vi "main.vi"() -> ()   [LabVIEW 2020]
doc: "This VI is used to talk with the psrr device and handle the errors produced by it."
uses:
  Typedef's/Last_Error_Details.ctl
  Typedef's/Q_Operations.ctl
  Typedef's/Q_State.ctl
  Typedef's/User_Events_Operations.ctl
  Typedef's/Data_Cluster.ctl
  Typedef's/Timer_Operations.ctl
  Typedef's/Error_Cluster.ctl
  Typedef's/PSRR_Value.ctl
  Typedef's/Error_Count.ctl
  Typedef's/Constants.ctl
  <vilib>/SLL Toolkit/SLL String/_SubVIs/I32 to String.vi
  <vilib>/SLL Toolkit/SLL String/SLL String.lvlib
panel:
  out "Last Error Details":T1
  out "Obtained PSRR":i32(graph)
  out "Table":string[][](table)
  in  "Error Log":bool
  out "Last Read PSRR (dB)":i32
  in  "Exit":bool
  in  "Wait Time (sec)":dbl=2.0 min=2.0
  out "Error?":bool
  out "Error Out":errorcluster
  in  "Error In":errorcluster
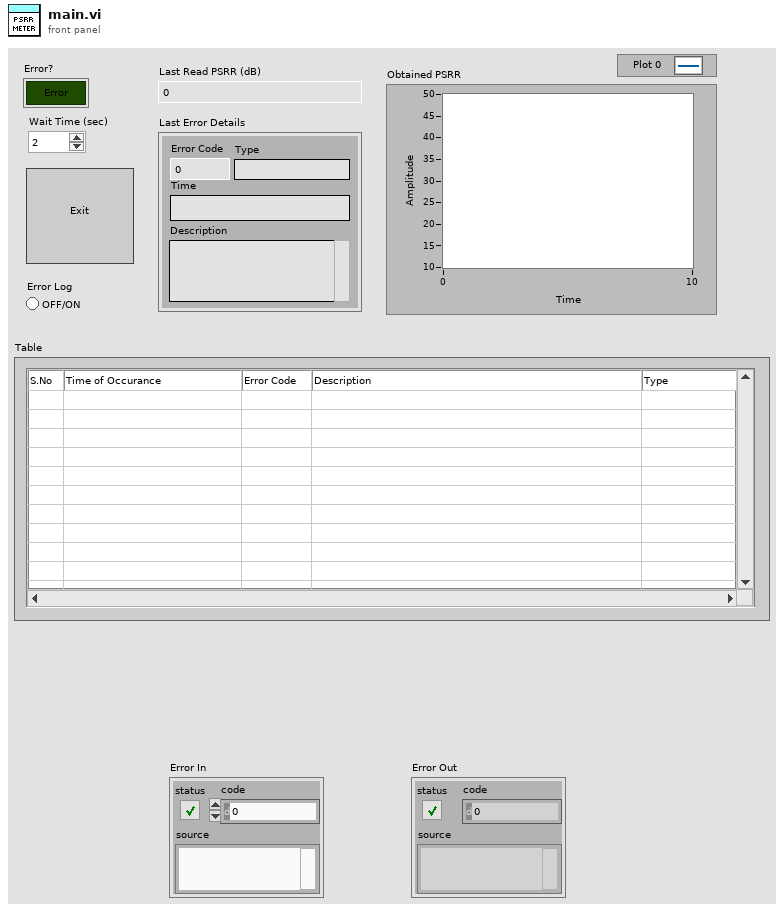
[diagram p1: front panel]
types:
  T1 = typedef "Last_Error_Details.ctl" = cluster{"Description":string, "Time":string, "Error Code":i32, "Type":string}
  T2 = typedef "Q_Operations.ctl" = enum16{"Create Q", "Enqueue", "Dequeue", "Enqueue N ele", "Enstack N ele", "Flush Q", "Destroy Q"}
  T3 = typedef "User_Events_Operations.ctl" = enum16{"Create", "Generate", "Destroy"}
  T4 = typedef "Q_State.ctl" = cluster{"State":string, "Data":variant}
  T5 = typedef "Data_Cluster.ctl" = cluster{"Wait Time":dbl, "Timer Operations":T6, "Error":T7, "Last Error Details":T1, "PSRR Value":T8, "Table Data":string[][], "Error Log?":bool, "Count":T9, "Constants":T10, "Data Folder Path":path}
  T6 = typedef "Timer_Operations.ctl" = cluster{"Prev Time":timestamp, "Set Time":timestamp}
  T7 = typedef "Error_Cluster.ctl" = errorcluster
  T8 = typedef "PSRR_Value.ctl" = cluster{"PSRR dB":i32, "PSRR Value Update?":bool}
  T9 = typedef "Error_Count.ctl" = cluster{"Passive Error":u8, "Unknown Error":u8, "S. No":i32}
  T10 = typedef "Constants.ctl" = cluster{"No Of Error":u8}
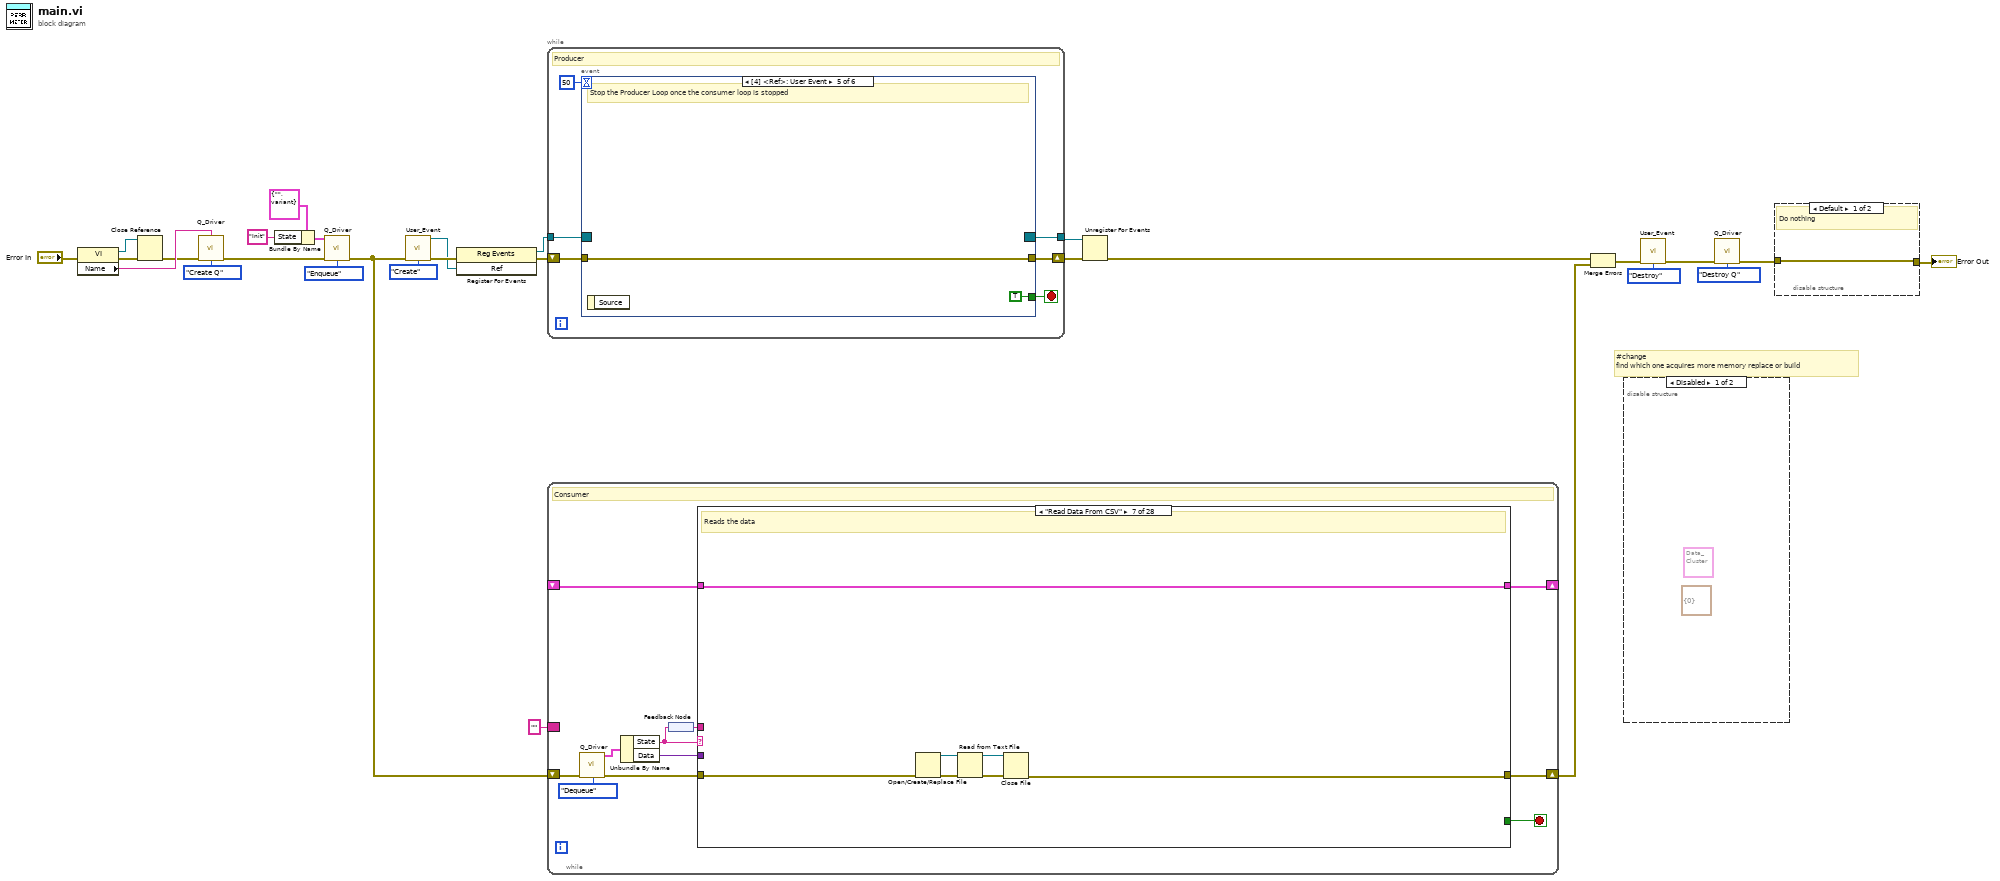
[diagram p0: block diagram]
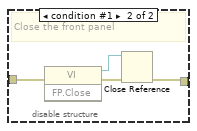
[diagram p3: hidden frame]
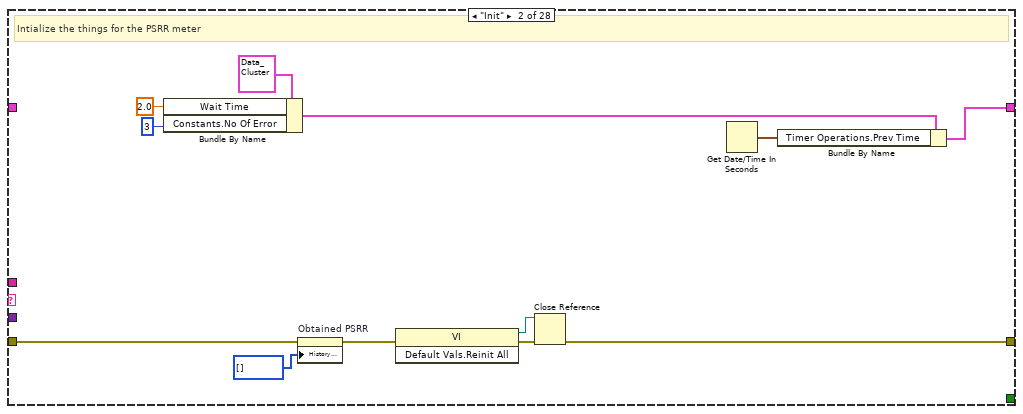
[diagram p5: hidden frame]
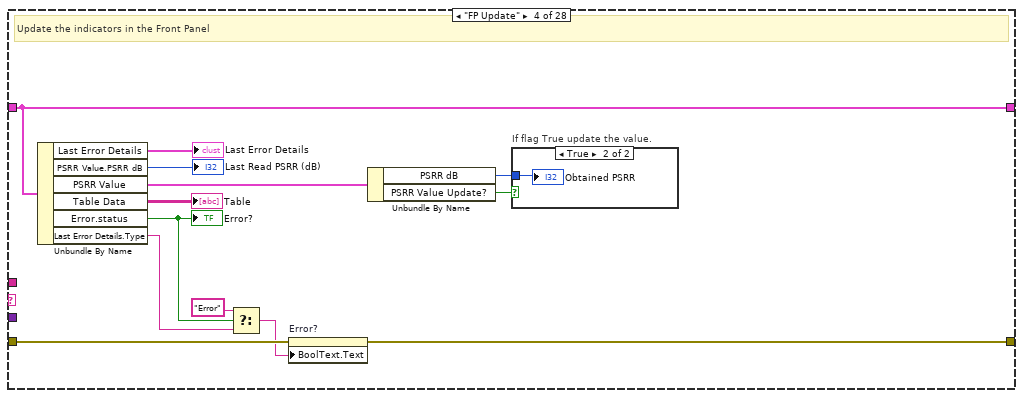
[diagram p7: hidden frame]
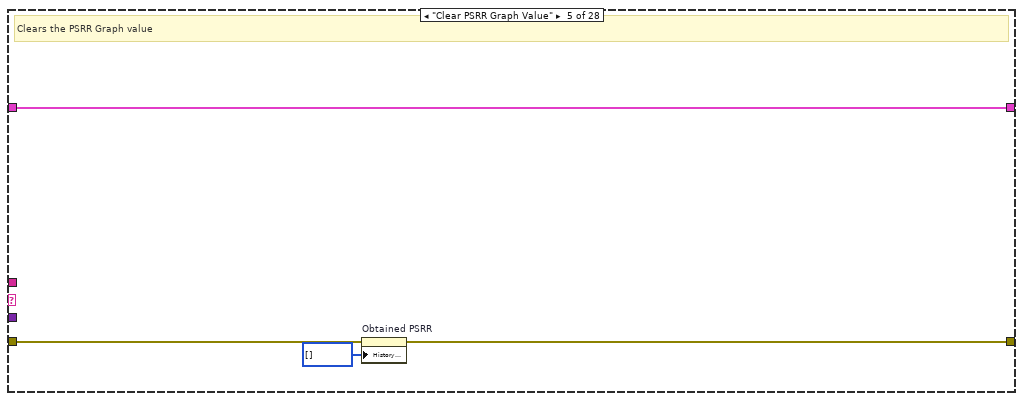
[diagram p9: hidden frame]
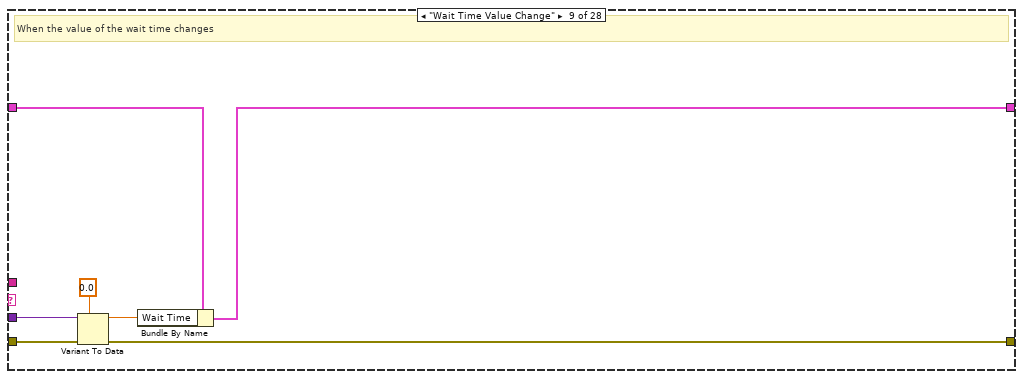
[diagram p12: hidden frame]
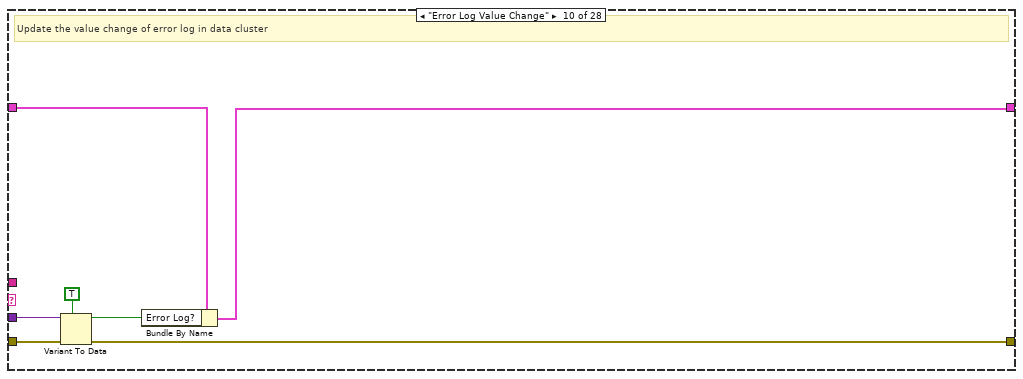
[diagram p13: hidden frame]
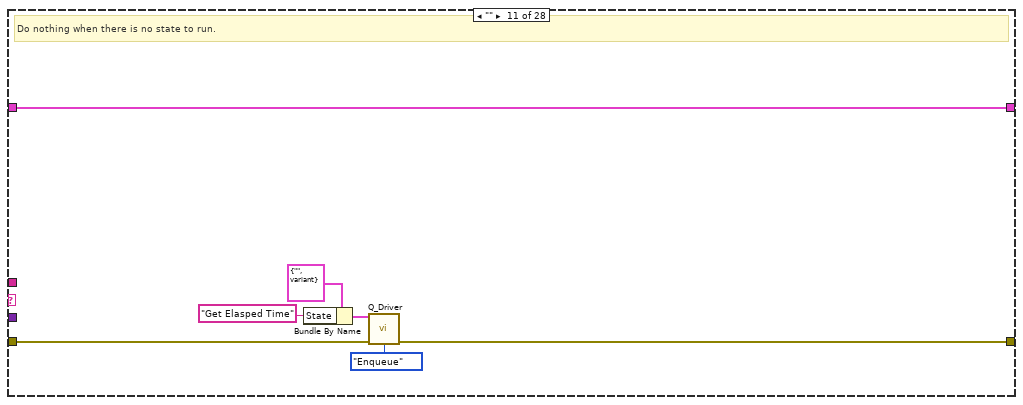
[diagram p14: hidden frame]
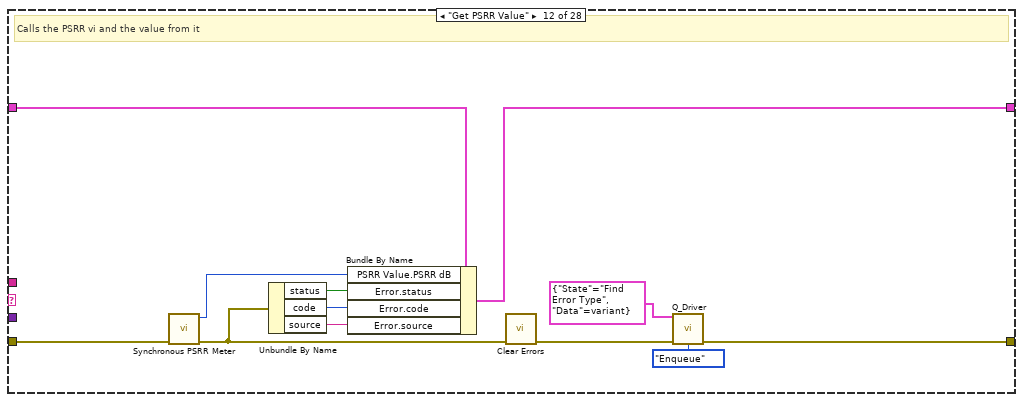
[diagram p15: hidden frame]
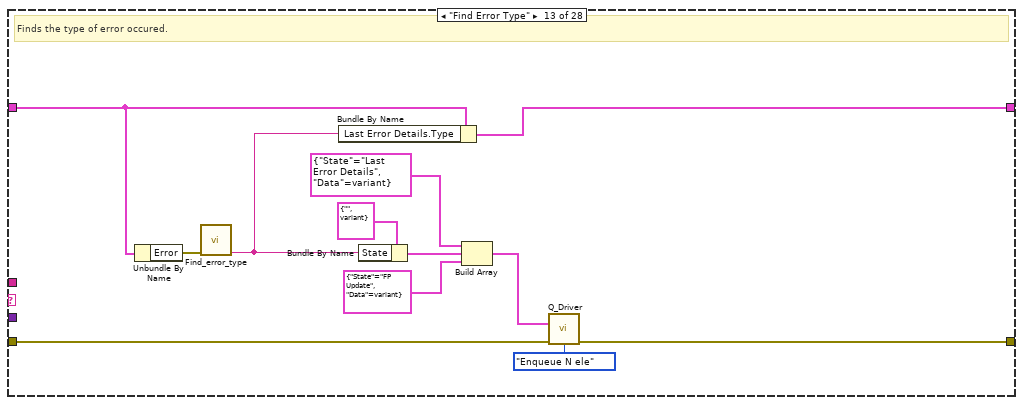
[diagram p16: hidden frame]
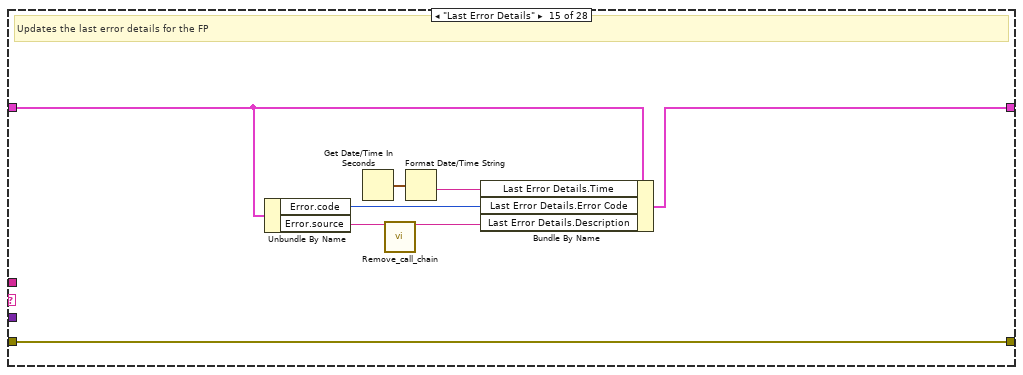
[diagram p18: hidden frame]
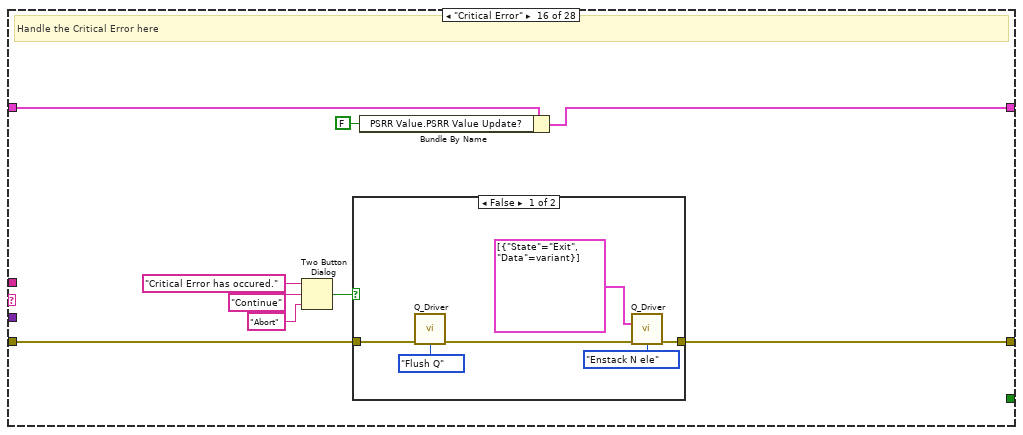
[diagram p19: hidden frame]
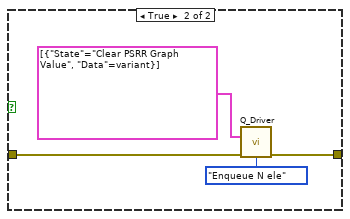
[diagram p20: hidden frame]
diagram:
  # "#change\nfind which one acquires more memory replace or build"
  n1 = property class="VI"(error in="Error In") -> (reference out=w5:refnum<vi>, error out=w24:errorcluster, "Name"=w23:string)  [unwired: 1 in]
  n2 = Close Reference(reference=w5, error in (no error)=w24) -> (error out=w21:errorcluster)
  n3 = call "Q_Driver.vi"("Q_Name"=w23, "Error In"=w21, "Operations"=Q_Operations."Create Q") -> ("Error Out"=w20:errorcluster)  [unwired: 11 in, 1 out]
  n4 = Bundle By Name(cluster=T4 {"State"="", "Data"=variant} ("State"), "State"="Init") -> (w15:T4)
  n5 = call "Q_Driver.vi"("State"=w15, "Error In"=w20, "Operations"=Q_Operations."Enqueue") -> ("Error Out"=w19:errorcluster)  [unwired: 11 in, 1 out]
  n6 = call "User_Event.vi"("Error In"=w19, "Enum"=User_Events_Operations."Create") -> ("Ref"=w11:refnum<user-event>, "Error Out"=w14:errorcluster)  [unwired: 12 in]
  n7 = register-events(error in=w14, w11) -> (reference out=w10:refnum<event-registration>, error out=w12:errorcluster)  [unwired: 1 in]
  n8 = while {
    shift-right: [w31] -> w28
    shift-left: w12 -> [w32]
    tunnel: w10 -> [w30]
    tunnel: [w29] -> w8
    stop <- w33 stop-if-true
    # "Producer"
    n9 = event shown="[4] <Ref>: User Event" {
      selector: w30 -> [_ _ _ _ _ _]
      dyn-events: [_ _ _ _ _ _] -> w29
      timeout: 50 -> [_ _ _ _ _ _]
      tunnel: [_ _ _ _ TRUE _] -> w33
      tunnel: w32 -> [w35 w36 w50 w55 w57 w58]
      tunnel: [w35 w43 w51 w54 w57 w59] -> w31
      event Timeout {
        # "When there is no event triggered."
        n10 = event-data() -> ()  [unwired: 1 in, 1 out]
      }
      event "Error Log": Value Change {
        # "When the error log is turned on"
        n11 = event-data() -> ("NewVal"=w39:bool)  [unwired: 1 in]
        n12 = To Variant(anything=w39) -> (Variant=w38:variant)
        n13 = Bundle By Name(cluster=T4 {"State"="", "Data"=variant} ("State"), "State"="Error Log Value Change", "Data"=w38) -> (w37:T4)
        n14 = call "Q_Driver.vi"("State"=w37, "Error In"=w36, "Operations"=Q_Operations."Enqueue") -> ("Error Out"=w43:errorcluster)  [unwired: 11 in, 1 out]
      }
      event "Wait Time (sec)": Value Change {
        # "When there is value change for error creation."
        n15 = event-data() -> ("NewVal"=w47:dbl)  [unwired: 1 in]
        n16 = To Variant(anything=w47) -> (Variant=w46:variant)
        n17 = Bundle By Name(cluster=T4 {"State"="", "Data"=variant} ("State"), "State"="Wait Time Value Change", "Data"=w46) -> (w44:T4)
        n18 = call "Q_Driver.vi"("State"=w44, "Error In"=w50, "Operations"=Q_Operations."Enqueue") -> ("Error Out"=w51:errorcluster)  [unwired: 11 in, 1 out]
      }
      event "Exit": Value Change {
        # "Exit the operation"
        n19 = event-data() -> ()  [unwired: 1 in, 1 out]
        n20 = call "Q_Driver.vi"("States[]"=T4[] [{"State"="Exit", "Data"=variant}], "Error In"=w55, "Operations"=Q_Operations."Enstack N ele") -> ("Error Out"=w54:errorcluster)  [unwired: 11 in, 1 out]
      }
      event User Event {
        # "Stop the Producer Loop once the consumer loop is stopped"
        n21 = event-data() -> ()  [unwired: 1 in, 1 out]
      }
      event Panel Close? {
        # "Handles the panel close event"
        n22 = event-data() -> ()  [unwired: 1 in, 1 out]
        n23 = call "Q_Driver.vi"("States[]"=T4[] [{"State"="Exit", "Data"=variant}], "Error In"=w58, "Operations"=Q_Operations."Enstack N ele") -> ("Error Out"=w59:errorcluster)  [unwired: 11 in, 1 out]
        n24 = event-data("Discard?"=TRUE) -> ()  [unwired: 1 in, 1 out]
      }
    }
  }
  n25 = while {
    shift-right: [w72] -> w26
    shift-left: w19 -> [w73]
    border: "" ("State") -> [_]
    shift-right: [w63] -> _
    shift-left: _ -> [w64]
    stop <- w65 stop-if-true
    # "Consumer"
    n26 = call "Q_Driver.vi"("Error In"=w73, "Operations"=Q_Operations."Dequeue") -> ("Dequeued State"=w70:T4, "Error Out"=w71:errorcluster)  [unwired: 12 in]
    n27 = Unbundle By Name(w70) -> ("State"=w67:string, "Data"=w69:variant)
    n28 = feedback-in #1(w67) -> ()
    n29 = feedback #1() -> (w66:string)
    n30 = case shown="\"Read Data From CSV\"" w67 {
      tunnel: w71 -> [w75 w79 w89 w102 w107 w109 w116 w118 w124 w132 w139 w150 w163 w165 w173 w182 w199 w220 w247 w269 w300 w302 w312 w324 w331 w333 w337 w355]
      tunnel: [w75 w78 w89 w94 w105 w109 w110 w118 w123 w129 w137 w142 w160 w165 w173 w177 w198 w220 w249 w272 w300 w302 w313 w324 w326 w333 w335 w355] -> w72
      tunnel: w69 -> [_ _ _ _ _ _ _ _ w122 w128 _ _ _ _ _ _ _ _ _ _ _ _ _ _ _ _ _ _]
      tunnel: w66 -> [_ _ _ _ _ _ _ _ _ _ _ _ _ _ _ _ _ _ _ _ _ _ _ _ _ _ w338 _]
      tunnel: [_ _ _ _ _ _ _ _ _ _ _ _ _ _ _ _ _ _ _ _ _ _ _ _ TRUE _ _ _] -> w65
      tunnel: [w74 w87 w88 w101 w106 w108 w115 w117 w125 w130 w138 w149 w157 w164 w167 w175 w202 w222 w244 w275 w298 w301 w311 w323 w329 w332 w346 w354] -> w63
      tunnel: w64 -> [w74 _ w88 w101 w106 w108 w115 w117 w121 w131 w138 w151 w162 w164 w166 w178 w200 w221 w243 w274 w299 w301 w310 w323 w329 w332 w346 w354]
      frame "/**** Initialization ****/" {
      }
      frame "Init" {
        # "Intialize the things for the PSRR meter"
        n31 = Bundle By Name(cluster=T5 {"Wait Time"=0.0, "Timer Operations"={"Prev Time"=timestamp(0 s since 1904-01-01), "Set Time"=timestamp(0 s since 1904-01-01)}, "Error"={"status"=FALSE, "code"=0, "source"=""}, "Last Error Details"={"Description"="", "Time"="", "Error Code"=0, "Type"=""}, "PSRR Value"={"PSRR dB"=0, "PSRR Value Update?"=FALSE}, "Table Data"=[], "Error Log?"=FALSE, "Count"={"Passive Error"=0, "Unknown Error"=0, "S. No"=1}, "Constants"={"No Of Error"=0}, "Data Folder Path"=path ""} ("Data Cluster"), "Wait Time"=2.0, "Constants.No Of Error"=3) -> (w83:T5)
        n32 = property on="Obtained PSRR" class="WFChart (strict)"(error in=w79, "History Data"=i32[] []) -> (error out=w82:errorcluster)  [unwired: 1 in, 1 out]
        n33 = invoke class="VI" method="Default Vals.Reinit All"(error in=w82) -> (reference out=w77:refnum<vi>, error out=w80:errorcluster)  [unwired: 2 in, 1 out]
        n34 = Close Reference(reference=w77, error in (no error)=w80) -> (error out=w78:errorcluster)
        n35 = Get Date/Time In Seconds() -> (seconds since 1Jan1904=w86:timestamp)
        n36 = Bundle By Name(cluster=w83, "Timer Operations.Prev Time"=w86) -> (w87:T5)
      }
      frame "/**** FP Related ****/" {
      }
      frame "FP Update" {
        # "Update the indicators in the Front Panel"
        n37 = Unbundle By Name(w101) -> ("Last Error Details"=→"Last Error Details":T1, "PSRR Value.PSRR dB"=→"Last Read PSRR (dB)":i32, "PSRR Value"=w98:T8, "Table Data"=→"Table":string[][], "Error.status"=w93:bool, "Last Error Details.Type"=w91:string)
        "Error?" <- w93
        n38 = Select(t="Error", s=w93, f=w91) -> (s? t:f=w90:string)
        n39 = property on="Error?" class="Bool (strict)"(error in=w102, "BoolText.Text"=w90) -> (error out=w94:errorcluster)  [unwired: 1 in, 1 out]
        n40 = Unbundle By Name(w98) -> ("PSRR dB"=w96:i32, "PSRR Value Update?"=w97:bool)
        n41 = case "If flag True update the value." shown="True" w97 {
          tunnel: w96 -> [_ w103]
          frame False {
          }
          frame True {
            "Obtained PSRR" <- w103
          }
        }
      }
      frame "Clear PSRR Graph Value" {
        # "Clears the PSRR Graph value"
        n42 = property on="Obtained PSRR" class="WFChart (strict)"(error in=w107, "History Data"=i32[] []) -> (error out=w105:errorcluster)  [unwired: 1 in, 1 out]
      }
      frame "/***** Configuration *****/" {
      }
      frame "Read Data From CSV" {
        # "Reads the data"
        n43 = Open/Create/Replace File(error in=w116) -> (refnum out=w113:refnum<file>, error out=w114:errorcluster)  [unwired: 5 in, 1 out]
        n44 = Read from Text File(file (use dialog)=w113, error in=w114) -> (refnum out=w111:refnum<file>, error out=w112:errorcluster)  [unwired: 2 in, 2 out]
        n45 = Close File(refnum=w111, error in=w112) -> (error out=w110:errorcluster)  [unwired: 1 out]
      }
      frame "/**** Functions ****/" {
      }
      frame "Wait Time Value Change" {
        # "When the value of the wait time changes"
        n46 = Variant To Data(error in=w124, type=0.0, Variant=w122) -> (data=w120:dbl, error out=w123:errorcluster)
        n47 = Bundle By Name(cluster=w121, "Wait Time"=w120) -> (w125:T5)
      }
      frame "Error Log Value Change" {
        # "Update the value change of error log in data cluster"
        n48 = Variant To Data(error in=w132, type=TRUE, Variant=w128) -> (data=w126:bool, error out=w129:errorcluster)
        n49 = Bundle By Name(cluster=w131, "Error Log?"=w126) -> (w130:T5)
      }
      frame "" {
        # "Do nothing when there is no state to run."
        n50 = Bundle By Name(cluster=T4 {"State"="", "Data"=variant} ("State"), "State"="Get Elasped Time") -> (w135:T4)
        n51 = call "Q_Driver.vi"("State"=w135, "Error In"=w139, "Operations"=Q_Operations."Enqueue") -> ("Error Out"=w137:errorcluster)  [unwired: 11 in, 1 out]
      }
      frame "Get PSRR Value" {
        # "Calls the PSRR vi and the value from it"
        n52 = call "Synchronous PSRR Meter.vi"("error in"=w150) -> ("error out"=w147:errorcluster, "PSRR (dB)"=w148:i32)  [unwired: 9 in]
        n53 = Unbundle By Name(w147) -> ("status"=w146:bool, "code"=w145:i32, "source"=w144:string)
        n54 = Bundle By Name(cluster=w151, "PSRR Value.PSRR dB"=w148, "Error.status"=w146, "Error.code"=w145, "Error.source"=w144) -> (w149:T5)
        n55 = call <vilib>:"Clear Errors.vi"("error in (no error)"=w147) -> ("error out"=w143:errorcluster)  [unwired: 5 in, 1 out]
        n56 = call "Q_Driver.vi"("State"=T4 {"State"="Find Error Type", "Data"=variant}, "Error In"=w143, "Operations"=Q_Operations."Enqueue") -> ("Error Out"=w142:errorcluster)  [unwired: 11 in, 1 out]
      }
      frame "Find Error Type" {
        # "Finds the type of error occured."
        n57 = Unbundle By Name(w162) -> ("Error"=w161:T7)
        n58 = call "Find_error_type.vi"("Error In"=w161) -> ("Error Type"=w156:string)  [unwired: 14 in]
        n59 = Bundle By Name(cluster=w162, "Last Error Details.Type"=w156) -> (w157:T5)
        n60 = Bundle By Name(cluster=T4 {"State"="", "Data"=variant} ("State"), "State"=w156) -> (w153:T4)
        n61 = Build Array(T4 {"State"="Last Error Details", "Data"=variant} ("State"), w153, T4 {"State"="FP Update", "Data"=variant} ("State")) -> (w155:T4[])
        n62 = call "Q_Driver.vi"("States[]"=w155, "Error In"=w163, "Operations"=Q_Operations."Enqueue N ele") -> ("Error Out"=w160:errorcluster)  [unwired: 11 in, 1 out]
      }
      frame "/***** PSRR Errors ****/" {
      }
      frame "Last Error Details" {
        # "Updates the last error details for the FP"
        n63 = Unbundle By Name(w166) -> ("Error.code"=w170:i32, "Error.source"=w169:string)
        n64 = Get Date/Time In Seconds() -> (seconds since 1Jan1904=w172:timestamp)
        n65 = call "Remove_call_chain.vi"("Error Description"=w169) -> ("Description Without Call Chain"=w168:string)  [unwired: 14 in]
        n66 = Format Date/Time String(seconds (now)=w172) -> (date/time string=w171:string)  [unwired: 2 in]
        n67 = Bundle By Name(cluster=w166, "Last Error Details.Time"=w171, "Last Error Details.Error Code"=w170, "Last Error Details.Description"=w168) -> (w167:T5)
      }
      frame "Critical Error" {
        # "Handle the Critical Error here"
        n68 = Two Button Dialog(message="Critical Error has occured.", 1:"Abort", 2:"Continue") -> (T button?=w176:bool)
        n69 = case shown="False" w176 {
          tunnel: w182 -> [w186 w192]
          tunnel: [w188 w191] -> w177
          frame False {
            n70 = call "Q_Driver.vi"("Error In"=w186, "Operations"=Q_Operations."Flush Q") -> ("Error Out"=w187:errorcluster)  [unwired: 12 in, 1 out]
            n71 = call "Q_Driver.vi"("States[]"=T4[] [{"State"="Exit", "Data"=variant}], "Error In"=w187, "Operations"=Q_Operations."Enstack N ele") -> ("Error Out"=w188:errorcluster)  [unwired: 11 in, 1 out]
          }
          frame True {
            n72 = call "Q_Driver.vi"("States[]"=T4[] [{"State"="Clear PSRR Graph Value", "Data"=variant}], "Error In"=w192, "Operations"=Q_Operations."Enqueue N ele") -> ("Error Out"=w191:errorcluster)  [unwired: 11 in, 1 out]
          }
        }
        n73 = Bundle By Name(cluster=w178, "PSRR Value.PSRR Value Update?"=FALSE) -> (w175:T5)
      }
      frame "Passive Error" {
        # "Handle the Passive Error here"
        n74 = Unbundle By Name(w200) -> ("Count.Passive Error"=w197:u8, "Constants.No Of Error"=w193:u8)
        n75 = Increment(x=w197) -> (x+1=w195:u8)
        n76 = Greater Or Equal?(x=w195, y=w193) -> (x >= y?=w196:bool)
        n77 = case shown="True" w196 {
          tunnel: w199 -> [w203 w208]
          tunnel: [w203 w207] -> w198
          tunnel: w195 -> [w204 _]
          tunnel: [w204 w205] -> w194
          frame False {
          }
          frame True {
            n78 = Two Button Dialog(message="Passive Error occured Three Times", 1:"Abort" ("F button name (\"Cancel\")"), 2:"Continue" ("T button name (\"OK\")")) -> (T button?=w206:bool)
            n79 = case shown="True" w206 {
              tunnel: w208 -> [w215 w219]
              tunnel: [w217 w219] -> w207
              tunnel: [_ u8 0] -> w205
              frame False {
                n80 = call "Q_Driver.vi"("Error In"=w215, "Operations"=Q_Operations."Flush Q") -> ("Error Out"=w216:errorcluster)  [unwired: 12 in, 1 out]
                n81 = call "Q_Driver.vi"("States[]"=T4[] [{"State"="Exit", "Data"=variant}], "Error In"=w216, "Operations"=Q_Operations."Enstack N ele") -> ("Error Out"=w217:errorcluster)  [unwired: 11 in, 1 out]
              }
              frame True {
              }
            }
          }
        }
        n82 = Bundle By Name(cluster=w200, "PSRR Value.PSRR Value Update?"=TRUE, "Count.Passive Error"=w194) -> (w202:T5)
      }
      frame "Warning" {
        # "Handle the Warnings here"
        n83 = Unbundle By Name(w221) -> ("Error Log?"=w223:bool)
        n84 = case shown="True" w223 {
          tunnel: w221 -> [w226 w240]
          tunnel: [w225 w239] -> w222
          frame False {
            # "If error log is false. Don't Update data in table"
            n85 = Bundle By Name(cluster=w226, "PSRR Value.PSRR Value Update?"=TRUE) -> (w225:T5)
          }
          frame True {
            # "Log the data in table"
            n86 = Unbundle By Name(w240) -> ("Count.S. No"=w237:i32, "Last Error Details.Time"=w235:string, "Last Error Details.Error Code"=w234:i32, "Last Error Details.Description"=w232:string, "Last Error Details.Type"=w231:string, "Table Data"=w229:string[][])
            n87 = call-poly <vilib>:"Number to String.vi"("Numeric"=w234) -> ("String"=w233:string)  [unwired: 10 in]
            n88 = call-poly <vilib>:"Number to String.vi"("Numeric"=w237) -> ("String"=w236:string)  [unwired: 10 in]
            n89 = Build Array(w236, w235, w233, w232, w231) -> (w230:string[])
            n90 = Increment(x=w237) -> (x+1=w238:i32)
            n91 = Build Array (concatenate)(w230, w229) -> (w228:string[][])
            n92 = Bundle By Name(cluster=w240, "Count.S. No"=w238, "Table Data"=w228, "PSRR Value.PSRR Value Update?"=TRUE) -> (w239:T5)
          }
        }
      }
      frame "Unknown Error" {
        # "Handle the Unknown Error here"
        n93 = call "Q_Driver.vi"("State"=T4 {"State"="Log Unknown Error", "Data"=variant}, "Error In"=w247, "Operations"=Q_Operations."Enqueue") -> ("Error Out"=w248:errorcluster)  [unwired: 11 in, 1 out]
        n94 = Unbundle By Name(w243) -> ("Count.Unknown Error"=w252:u8, "Constants.No Of Error"=w241:u8)
        n95 = Increment(x=w252) -> (x+1=w251:u8)
        n96 = Greater Or Equal?(x=w251, y=w241) -> (x >= y?=w250:bool)
        n97 = case shown="False" w250 {
          tunnel: w251 -> [w253 _]
          tunnel: w248 -> [w254 w258]
          tunnel: [w254 w257] -> w249
          tunnel: [w253 u8 0] -> w242
          frame False {
            # "Just increase the count"
          }
          frame True {
            # "When the count is greater than three"
            n98 = Two Button Dialog(message="Unknown Error occured more than 3 times", 1:"Abort" ("F button name (\"Cancel\")"), 2:"Continue" ("T button name (\"OK\")")) -> (T button?=w256:bool)
            n99 = case shown="False" w256 {
              tunnel: [w264 w268] -> w257
              tunnel: w258 -> [w267 w268]
              frame False {
                # "Abort the VI"
                n100 = call "Q_Driver.vi"("Error In"=w267, "Operations"=Q_Operations."Flush Q") -> ("Error Out"=w265:errorcluster)  [unwired: 12 in, 1 out]
                n101 = call "Q_Driver.vi"("States[]"=T4[] [{"State"="Exit", "Data"=variant}], "Error In"=w265, "Operations"=Q_Operations."Enstack N ele") -> ("Error Out"=w264:errorcluster)  [unwired: 11 in, 1 out]
              }
              frame True {
                # "Continue the operation do nothing"
              }
            }
          }
        }
        n102 = Bundle By Name(cluster=w243, "Count.Unknown Error"=w242) -> (w244:T5)
      }
      frame "Log Unknown Error" {
        # "Logs the data for unknown error"
        n103 = Unbundle By Name(w274) -> ("Error Log?"=w273:bool)
        n104 = case shown="True" w273 {
          tunnel: w274 -> [w278 w285]
          tunnel: [w276 w286] -> w275
          frame False {
            # "Don't Update the data in graph"
            n105 = Bundle By Name(cluster=w278, "PSRR Value.PSRR Value Update?"=FALSE) -> (w276:T5)
          }
          frame True {
            # "Log the data into the table."
            n106 = Unbundle By Name(w285) -> ("Count.S. No"=w295:i32, "Last Error Details.Time"=w293:string, "Last Error Details.Error Code"=w292:i32, "Last Error Details.Type"=w291:string, "Table Data"=w289:string[][], "Error.source"=w283:string)
            n107 = call-poly <vilib>:"Number to String.vi"("Numeric"=w292) -> ("String"=w284:string)  [unwired: 10 in]
            n108 = Match Pattern(string=w283, regular expression="<APPEND>") -> (before substring=w280:string)  [unwired: 1 in, 3 out]
            n109 = call-poly <vilib>:"Number to String.vi"("Numeric"=w295) -> ("String"=w294:string)  [unwired: 10 in]
            n110 = Concatenate Strings(w284, "-" ("string"), w280) -> (w279:string)
            n111 = Increment(x=w295) -> (x+1=w296:i32)
            n112 = Build Array(w294, w293, w284, w279, w291) -> (w290:string[])
            n113 = Build Array (concatenate)(w290, w289) -> (w288:string[][])
            n114 = Bundle By Name(cluster=w285, "Count.S. No"=w296, "Table Data"=w288, "PSRR Value.PSRR Value Update?"=FALSE, "Last Error Details.Description"=w279) -> (w286:T5)
          }
        }
        n115 = call "Q_Driver.vi"("State"=T4 {"State"="FP Update", "Data"=variant}, "Error In"=w269, "Operations"=Q_Operations."Enqueue") -> ("Error Out"=w272:errorcluster)  [unwired: 11 in, 1 out]
      }
      frame "No Error" {
        # "When there is no error"
        n116 = Bundle By Name(cluster=w299, "PSRR Value.PSRR Value Update?"=TRUE) -> (w298:T5)
      }
      frame "/***** Timer Operations ****/" {
      }
      frame "Get Elasped Time" {
        # "Gets the elapsed time from the start time."
        n117 = Unbundle By Name(w310) -> ("Timer Operations.Prev Time"=w309:timestamp, "Wait Time"=w306:dbl)
        n118 = Get Date/Time In Seconds() -> (seconds since 1Jan1904=w308:timestamp)
        n119 = To Double Precision Float(number=w309) -> (double precision float=w305:dbl)
        n120 = To Double Precision Float(number=w308) -> (double precision float=w304:dbl)
        n121 = Subtract(x=w304, y=w305) -> (x-y=w303:dbl)
        n122 = Greater?(x=w303, y=w306) -> (0:w307:bool)
        n123 = case shown="True" w307 {
          tunnel: w312 -> [w315 w321]
          tunnel: [w315 w322] -> w313
          tunnel: w310 -> [w314 w318]
          tunnel: [w314 w317] -> w311
          frame False {
          }
          frame True {
            # "Set point is reached."
            n124 = Get Date/Time In Seconds() -> (seconds since 1Jan1904=w316:timestamp)
            n125 = Bundle By Name(cluster=w318, "Timer Operations.Prev Time"=w316) -> (w317:T5)
            n126 = call "Q_Driver.vi"("State"=T4 {"State"="Get PSRR Value", "Data"=variant}, "Error In"=w321, "Operations"=Q_Operations."Enqueue") -> ("Error Out"=w322:errorcluster)  [unwired: 11 in, 1 out]
          }
        }
      }
      frame "/**** Exit ****/" {
      }
      frame "Exit" {
        # "Exit the process"
        n127 = call "User_Event.vi"("Error In"=w331, "Enum"=User_Events_Operations."Generate") -> ("Error Out"=w328:errorcluster)  [unwired: 12 in, 1 out]
        n128 = call "Q_Driver.vi"("Error In"=w328, "Operations"=Q_Operations."Flush Q") -> ("Error Out"=w326:errorcluster)  [unwired: 12 in, 1 out]
      }
      frame "/**** Error States ****/" {
      }
      frame "Error" {
        # "Handle the errors here."
        n129 = Unbundle By Name(w337) -> ("code"=w341:i32, "source"=w342:string)
        n130 = call <vilib>:"Clear Errors.vi"("error in (no error)"=w337, "specific error code to clear (0: all)"=w341) -> ("error out"=w339:errorcluster)  [unwired: 4 in, 1 out]
        n131 = Format Into String(format string="Error occurred in state \"%s\"!!\nError Code: %d\nError Source: %s\n\nDo you wish to continue?", error in=w339, w338, w341, w342) -> (resulting string=w343:string, error out=w336:errorcluster)  [unwired: 1 in]
        n132 = Two Button Dialog(message=w343, 1:"Exit" ("F button name (\"Cancel\")"), 2:"Continue" ("T button name (\"OK\")")) -> (T button?=w334:bool)
        n133 = case shown="True" w334 {
          tunnel: [w347 w352] -> w335
          tunnel: w336 -> [w347 w353]
          frame False {
          }
          frame True {
            n134 = call "Q_Driver.vi"("Error In"=w353, "Operations"=Q_Operations."Flush Q") -> ("Error Out"=w349:errorcluster)  [unwired: 12 in, 1 out]
            n135 = call "Q_Driver.vi"("State"=T4 {"State"="Exit", "Data"=variant}, "Error In"=w349, "Operations"=Q_Operations."Enqueue") -> ("Error Out"=w352:errorcluster)  [unwired: 11 in, 1 out]
          }
        }
      }
      frame "Developer Error", Default {
        # "When there is some mistake made by developer"
      }
    }
  }
  n136 = Unregister For Events(event registration refnum=w8, error in=w28) -> (error out=w9:errorcluster)
  n137 = Merge Errors(w9, w26) -> (w27:errorcluster)
  n138 = disable-structure shown="Disabled" {
    frame Disabled {
      (unwired) T10 {"No Of Error"=0} ("Constants")
      (unwired) T5 {"Wait Time"=0.0, "Timer Operations"={"Prev Time"=timestamp(0 s since 1904-01-01), "Set Time"=timestamp(0 s since 1904-01-01)}, "Error"={"status"=FALSE, "code"=0, "source"=""}, "Last Error Details"={"Description"="", "Time"="", "Error Code"=0, "Type"=""}, "PSRR Value"={"PSRR dB"=0, "PSRR Value Update?"=FALSE}, "Table Data"=[], "Error Log?"=FALSE, "Count"={"Passive Error"=0, "Unknown Error"=0, "S. No"=0}, "Constants"={"No Of Error"=0}, "Data Folder Path"=path ""} ("Data Cluster")
    }
    frame Enabled {
    }
  }
  n139 = call "User_Event.vi"("Error In"=w27, "Enum"=User_Events_Operations."Destroy") -> ("Error Out"=w3:errorcluster)  [unwired: 12 in, 1 out]
  n140 = call "Q_Driver.vi"("Error In"=w3, "Operations"=Q_Operations."Destroy Q") -> ("Error Out"=w2:errorcluster)  [unwired: 12 in, 1 out]
  n141 = disable-structure shown="Default" {
    disable-tunnel: [w356 w358] -> w4
    disable-tunnel: w2 -> [w356 w360]
    frame condition #0 (active) {
      # "Do nothing"
    }
    frame condition #1 {
      # "Close the front panel"
      n142 = invoke class="VI" method="FP.Close"(error in=w360) -> (reference out=w357:refnum<vi>, error out=w359:errorcluster)  [unwired: 2 in, 1 out]
      n143 = Close Reference(reference=w357, error in (no error)=w359) -> (error out=w358:errorcluster)
    }
  }
  "Error Out" <- w4
